vi "Handle Last Ack Core.vi"(4 "error in (no error)":errorcluster, 6 "Last Ack":refnum<class "Last Ack.lvclass">, 7 "Logger Mananger in":refnum<class "Logger Mananger.lvclass">) -> (0 "error out":errorcluster, 3 "Logger Mananger out":refnum<class "Logger Mananger.lvclass">)   [LabVIEW 2020, in "Logging.lvlib" / "Logger Mananger.lvclass"]
doc: "(<B>Filename</B>: Actor Framework.lvlib:Actor.lvclass:Handle Last Ack Core.vi)\n\nDefines how the caller actor responds to the Last Ack message from a nested actor. The Last Ack message is the final message a nested actor sends to its caller before it shuts down. The message contains information about the final state of the nested actor.\n\nBy default, this method does nothing except return any error the nested actor sent. A descendant class may override this method to define behavior."
uses:
  Logger Mananger.lvclass
  <vilib>/ActorFramework/LastAck/Last Ack.lvclass
  Logger Mananger.lvclass/Logger Mananger.ctl
  <vilib>/ActorFramework/Actor/Actor.lvclass
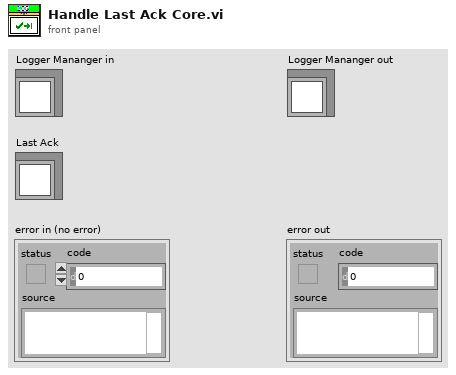
[diagram p1: front panel]
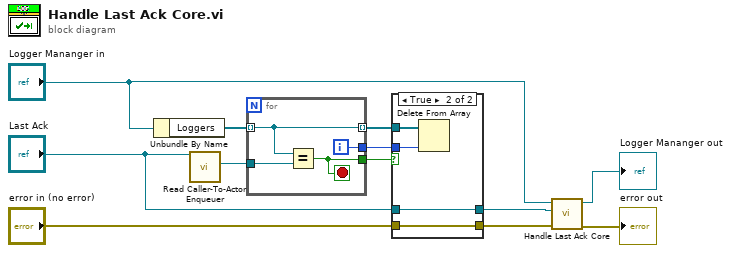
[diagram p0: block diagram]
diagram:
  n1 = Unbundle By Name("Logger Mananger in") -> ("Loggers"=w9:refnum<class "Message Enqueuer.lvclass">[])
  n2 = call <vilib>:"Read Caller-To-Actor Enqueuer.vi"("Last Ack"="Last Ack") -> ("Caller-to-Actor Enqueuer"=w8:refnum<class "Message Enqueuer.lvclass">)  [unwired: 10 in]
  n3 = for {
    tunnel: w9 -> [w14] mode=indexing
    tunnel: w8 -> [w16]
    tunnel: [w15] -> w7
    tunnel: [w14] -> w6 mode=indexing
    tunnel: [w13] -> w5
    i -> [w13]
    stop <- w15 stop-if-true
    n4 = Equal?(x=w14, y=w16) -> (x = y?=w15:bool)
  }
  n5 = case shown="True" w7 {
    tunnel: w6 -> [_ w22]
    tunnel: w5 -> [_ w21]
    tunnel: [w18 w20] -> w4
    tunnel: "Last Ack" -> [w18 w20]
    tunnel: "error in (no error)" -> [w17 w19]
    tunnel: [w17 w19] -> w1
    frame False {
    }
    frame True {
      n6 = Delete From Array(array=w22, index=w21) -> ()  [unwired: 1 in, 2 out]
    }
  }
  n7 = call-parent "Handle Last Ack Core.vi"("error in (no error)"=w1, "Last Ack"=w4, "Actor in"="Logger Mananger in") -> ("error out"=→"error out":errorcluster, "Actor out"=→"Logger Mananger out":refnum<class "Logger Mananger.lvclass">)  [unwired: 3 in]
